vi "BRig_Host_dataRunState_dataTS_nTrial.vi"() -> (2 "output_idx_dataTS_nTrial":i32)   [LabVIEW 2014]
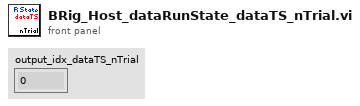
[diagram p1: front panel]
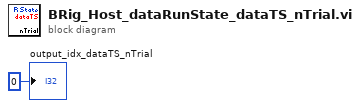
[diagram p0: block diagram]
diagram:
  "output_idx_dataTS_nTrial" <- 0 ("output_idx_dataTS")
